vi "Connect.vi"(8 "error in (no error)":errorcluster, 10 "Channel(s)":string, 11 "Hioki 9002 in":refnum<class "Hioki 9002.lvclass">) -> (0 "error out":errorcluster, 3 "Hioki 9002 out":refnum<class "Hioki 9002.lvclass">)   [LabVIEW 2025, in "Switch.lvlib" / "Hioki 9002.lvclass"]
uses:
  Hioki 9002.lvclass
  Hioki 9002.lvclass/Hioki 9002.ctl
  <instrlib>/HIOKI SW100X Series/HIOKI SW100X Series.lvlib
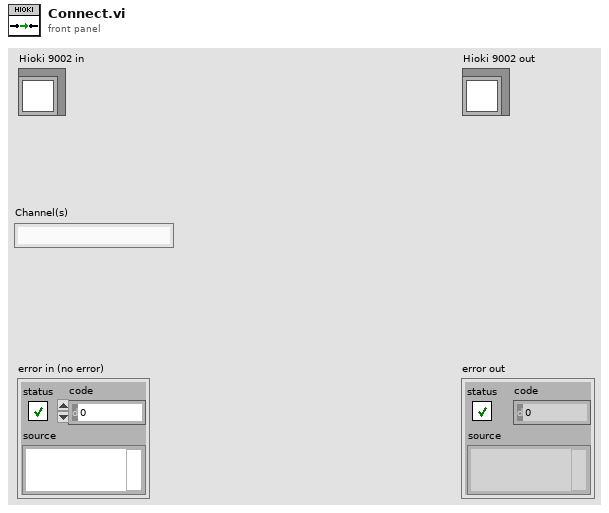
[diagram p1: front panel]
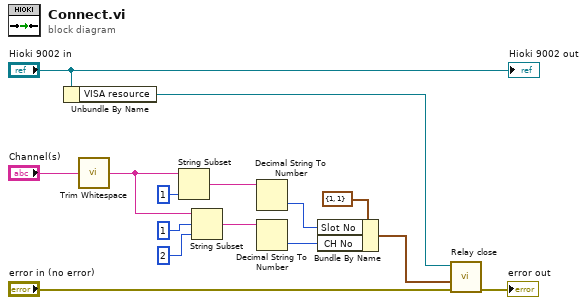
[diagram p0: block diagram]
diagram:
  n1 = Unbundle By Name("Hioki 9002 in") -> ("VISA resource"=w1:refnum<visa-resource-name>)
  n2 = call <vilib>:"Trim Whitespace.vi"("string"="Channel(s)") -> ("trimmed string"=w13:string)  [unwired: 1 in]
  n3 = String Subset(string=w13, length (rest)=1 ("length (rest)")) -> (substring=w12:string)  [unwired: 1 in]
  n4 = String Subset(string=w13, offset (0)=1, length (rest)=2 ("length (rest)")) -> (substring=w15:string)
  n5 = Decimal String To Number(string=w12) -> (number=w8:i32)  [unwired: 2 in, 1 out]
  n6 = Decimal String To Number(string=w15) -> (number=w9:i32)  [unwired: 2 in, 1 out]
  n7 = Bundle By Name(cluster=cluster{"Slot No":u16, "CH No":u16} {"Slot No"=1, "CH No"=1} ("Close Point"), "Slot No"=w8, "CH No"=w9) -> (w7:cluster{"Slot No":u16, "CH No":u16})
  n8 = call <instrlib>:"Relay close.vi"("error in"="error in (no error)", "Close Point"=w7, "VISA resource name"=w1) -> ("error out"=→"error out":errorcluster)  [unwired: 6 in, 2 out]
  "Hioki 9002 out" <- "Hioki 9002 in"
